vi "Create Table.vi"(3 "error in (no error)":errorcluster, 4 "column information":T1[](array[typedef]), 5 "table":string) -> (0 "error out":errorcluster)   [LabVIEW 2023]
uses:
  <vilib>/addons/database/Auxilliary.llb/DB Tools Column Info.ctl
  <vilib>/addons/database/Auxilliary.llb/DB Tools DataTypes.ctl
  <vilib>/addons/database/Connection.llb/DB Tools Open Connec (String).vi
  <vilib>/addons/database/NI_Database_API.lvlib
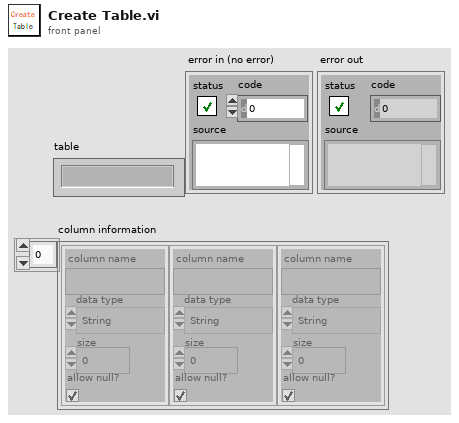
[diagram p1: front panel]
types:
  T1 = typedef "NI_Database_API.lvlib/DB Tools Column Info.ctl" = cluster{"column name":string, "data type":T2, "size":i32, "allow null?":bool}
  T2 = typedef "NI_Database_API.lvlib/DB Tools DataTypes.ctl" = enum16{"String", "Long (I32)", "Single (SGL)", "Double (DBL)", "Date/Time", "Binary"}
  T3 = typedef "NI_Database_API.lvlib/Conn ObjectReference.ctl" = refnum<k1>
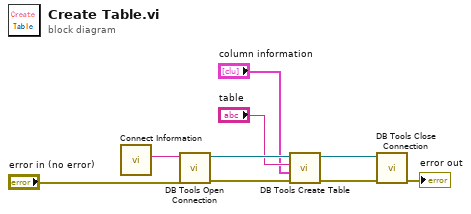
[diagram p0: block diagram]
diagram:
  n1 = call "Connect Information.vi"() -> ("Connect Info"=w9:string)  [unwired: 11 in]
  n2 = call-poly <vilib>:"DB Tools Open Connection.vi"("error in (no error)"="error in (no error)", "connection information"=w9) -> ("error out"=w7:errorcluster, "connection reference"=w8:T3)  [unwired: 6 in]
  n3 = call <vilib>:"DB Tools Create Table.vi"("error in (no error)"=w7, "column information"="column information", "table"="table", "connection reference"=w8) -> ("error out"=w3:errorcluster, "connection reference out"=w4:T3)  [unwired: 4 in]
  n4 = call <vilib>:"DB Tools Close Connection.vi"("error in (no error)"=w3, "connection reference"=w4) -> ("error out"=→"error out":errorcluster)  [unwired: 5 in]
